vi "Part 2.vi"(11 "Input":string) -> (3 "Output":i64)   [LabVIEW 2021]
uses:
  <userlib>/_OpenG.lib/string/string.llb/Convert EOLs (String)__ogtk.vi
panel:
  out "concatenated string":string
  out "Array":string[](array[string])
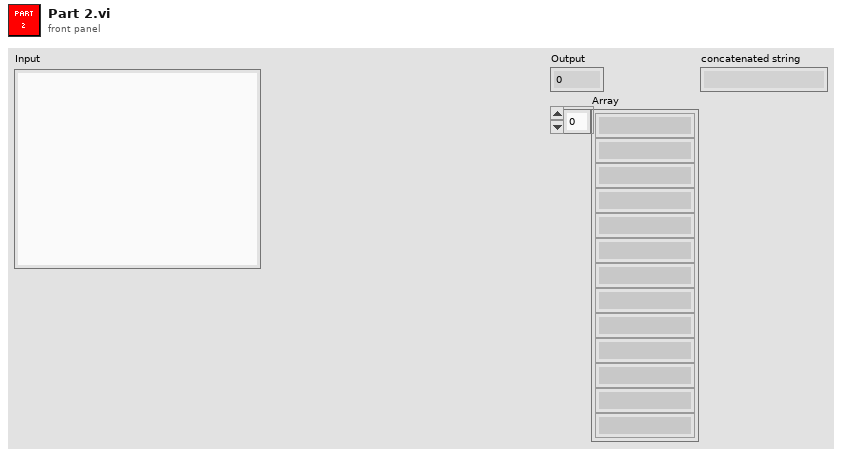
[diagram p1: front panel]
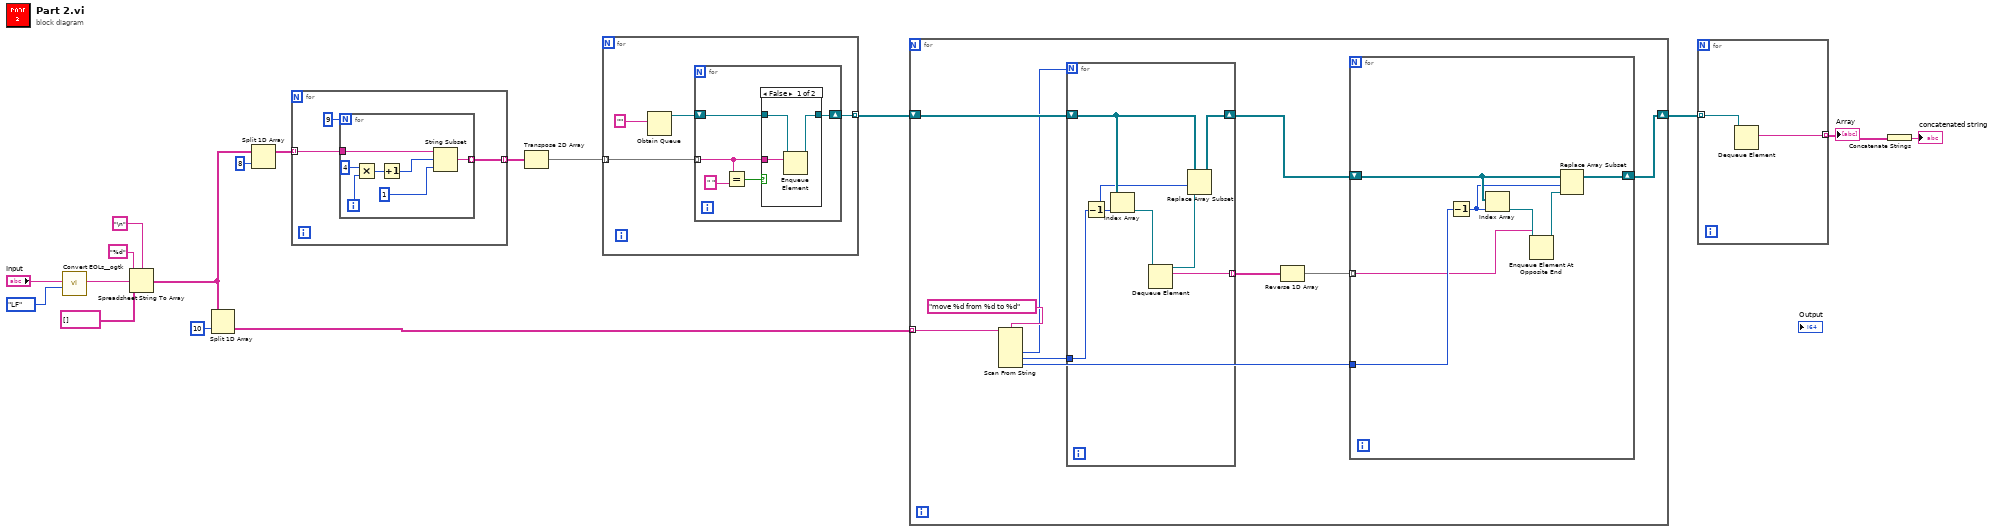
[diagram p0: block diagram]
diagram:
  n1 = call-poly <userlib>:"Convert EOLs__ogtk.vi"("Convert to:"=enum16{"CR", "LF", "CRLF"}."LF", "String in"="Input") -> ("String out"=w14:string)  [unwired: 9 in]
  n2 = Spreadsheet String To Array(delimiter (Tab)="\n", format string="%d", spreadsheet string=w14, array type (2D Dbl)=string[] []) -> (array=w10:string[])
  n3 = Split 1D Array(array=w10, index=10) -> (second subarray=w6:string[])  [unwired: 1 out]
  n4 = Split 1D Array(array=w10, index=8) -> (first subarray=w9:string[])  [unwired: 1 out]
  n5 = for {
    tunnel: w9 -> [w20] mode=indexing
    tunnel: [w18] -> w8 mode=indexing
    n6 = for {
      N: 9 -> [_]
      tunnel: w20 -> [w27]
      tunnel: [w24] -> w18 mode=indexing
      i -> [w26]
      n7 = Multiply(x=4, y=w26) -> (x*y=w23:i32)
      n8 = Increment(x=w23) -> (x+1=w22:i32)
      n9 = String Subset(string=w27, offset (0)=w22, length (rest)=1 ("length (rest)")) -> (substring=w24:string)
    }
  }
  n10 = Transpose 2D Array(2D array=w8) -> (transposed array=w7:string[][])
  n11 = for {
    tunnel: w7 -> [w30] mode=indexing
    tunnel: [w28] -> w5 mode=indexing
    n12 = Obtain Queue(element data type="") -> (queue out=w29:refnum<queue>)  [unwired: 4 in, 2 out]
    n13 = for {
      tunnel: w30 -> [w33] mode=indexing
      shift-right: [w35] -> w28
      shift-left: w29 -> [w36]
      n14 = Equal?(x=w33, y=" ") -> (x = y?=w34:bool)
      n15 = case shown="False" w34 {
        tunnel: w36 -> [w39 w40]
        tunnel: [w38 w40] -> w35
        tunnel: w33 -> [w37 _]
        frame False {
          n16 = Enqueue Element(queue=w39, element=w37) -> (queue out=w38:refnum<queue>)  [unwired: 2 in, 2 out]
        }
        frame True {
        }
      }
    }
  }
  n17 = for {
    tunnel: w6 -> [w50] mode=indexing
    shift-right: [w45] -> w4
    shift-left: w5 -> [w48]
    n18 = Scan From String(format string="move %d from %d to %d", input string=w50) -> (output 1=w42:i32, output 2=w47:i32, output 3=w46:i32)  [unwired: 5 in, 3 out]
    n19 = for {
      N: w42 -> [_]
      tunnel: w47 -> [w63]
      tunnel: [w59] -> w43 mode=indexing
      shift-right: [w58] -> w44
      shift-left: w48 -> [w64]
      n20 = Decrement(x=w63) -> (x-1=w60:i32)
      n21 = Index Array(array=w64, index=w60) -> (element=w62:refnum<queue>)
      n22 = Dequeue Element(queue=w62) -> (queue out=w61:refnum<queue>, element=w59:string)  [unwired: 2 in, 2 out]
      n23 = Replace Array Subset(array=w64, new element=w61, index=w60) -> (w58:refnum<queue>[])
    }
    n24 = Reverse 1D Array(array=w43) -> (reversed array=w41:string[])
    n25 = for {
      tunnel: w46 -> [w57]
      tunnel: w41 -> [w51] mode=indexing
      shift-right: [w56] -> w45
      shift-left: w44 -> [w54]
      n26 = Decrement(x=w57) -> (x-1=w52:i32)
      n27 = Index Array(array=w54, index=w52) -> (element=w55:refnum<queue>)
      n28 = Enqueue Element At Opposite End(queue=w55, element=w51) -> (queue out=w53:refnum<queue>)  [unwired: 2 in, 2 out]
      n29 = Replace Array Subset(array=w54, new element=w53, index=w52) -> (w56:refnum<queue>[])
    }
  }
  n30 = for {
    tunnel: w4 -> [w66] mode=indexing
    tunnel: [w65] -> w3 mode=indexing
    n31 = Dequeue Element(queue=w66) -> (element=w65:string)  [unwired: 2 in, 3 out]
  }
  "Array" <- w3
  n32 = Concatenate Strings(w3) -> (→"concatenated string":string)
